vi "力特性 回正率.vi"(8 "油压B":dbl[](array[numeric]), 9 "油压A":dbl[](array[numeric]), 10 "扭矩B":dbl[](array[numeric]), 11 "扭矩A":dbl[](array[numeric])) -> (3 "回正率":dbl)   [LabVIEW 2015, in "Logging.lvlib"]
uses:
  Logging.lvlib
  <vilib>/Analysis/1siggen.llb/Ramp Pattern by Samples.vi
  <vilib>/gmath/NI_Gmath.lvlib
  <vilib>/Analysis/NI_AALBase.lvlib
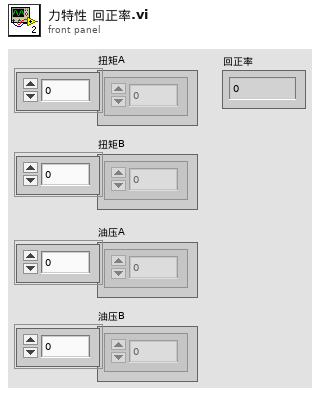
[diagram p1: front panel]
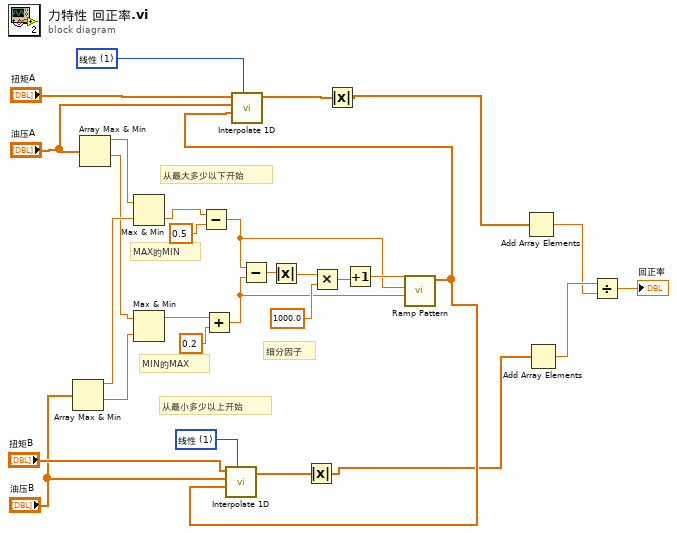
[diagram p0: block diagram]
diagram:
  w14 = 1 items=["最近", "线性", "样条", "cubic Hermite", "拉格朗日"] ("method")
  w29 = 1 items=["最近", "线性", "样条", "cubic Hermite", "拉格朗日"] ("method")
  # "细分因子"
  # "从最大多少以下开始"
  # "从最小多少以上开始"
  # "MIN的MAX"
  # "MAX的MIN"
  n1 = Array Max & Min(array="油压B") -> (max value=w27:dbl, min value=w25:dbl)  [unwired: 2 out]
  n2 = Array Max & Min(array="油压A") -> (max value=w28:dbl, min value=w26:dbl)  [unwired: 2 out]
  n3 = Max & Min(x=w28, y=w27) -> (min(x,y)=w8:dbl)  [unwired: 1 out]
  n4 = Max & Min(x=w26, y=w25) -> (max(x,y)=w9:dbl)  [unwired: 1 out]
  n5 = Subtract(x=w8, y=0.5) -> (x-y=w17:dbl)
  n6 = Add(x=w9, y=0.2) -> (x+y=w16:dbl)
  n7 = Subtract(x=w17, y=w16) -> (x-y=w22:dbl)
  n8 = Absolute Value(x=w22) -> (abs(x)=w20:dbl)
  n9 = Multiply(x=w20, y=1000.0) -> (x*y=w21:dbl)
  n10 = Increment(x=w21) -> (x+1=w18:dbl)
  n11 = call-poly <vilib>:"Ramp Pattern.vi"("start"=w16, "end"=w17, "samples"=w18) -> ("Ramp Pattern"=w15:dbl[])  [unwired: 7 in, 1 out]
  n12 = call <vilib>:"Interpolate 1D.vi"("method"=w14, "xi"=w15, "X"="油压B", "Y"="扭矩B") -> ("yi"=w4:dbl[])  [unwired: 5 in, 2 out]
  n13 = call <vilib>:"Interpolate 1D.vi"("method"=w29, "xi"=w15, "X"="油压A", "Y"="扭矩A") -> ("yi"=w6:dbl[])  [unwired: 5 in, 2 out]
  n14 = Absolute Value(x=w4) -> (abs(x)=w3:dbl[])
  n15 = Absolute Value(x=w6) -> (abs(x)=w5:dbl[])
  n16 = Add Array Elements(numeric array=w5) -> (sum=w1:dbl)
  n17 = Add Array Elements(numeric array=w3) -> (sum=w2:dbl)
  n18 = Divide(x=w2, y=w1) -> (x/y=→"回正率":dbl)
